vi "ReadATEQData.vi"(11 "Chaîne":string) -> (0 "Prg number":string, 1 "Valeur":i32, 2 "result":string, 3 "Status":string)   [LabVIEW 2020]
uses:
  <vilib>/regexp/Match Regular Expression.xnode
panel:
  # "<20>:(AL):PRESSION HAUTE\n<30>:(DR):-126 Pa\n<30>:(DT):2 Pa\n<30>:(DR):-10 Pa\n<30>:(PB):1 Pa\n<30>:(PB):1 Pa\n<30>:(PB):-2 Pa\n<30>:(DR):-197 Pa\n^C"
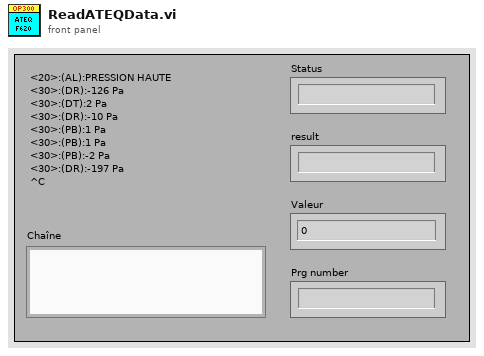
[diagram p1: front panel]
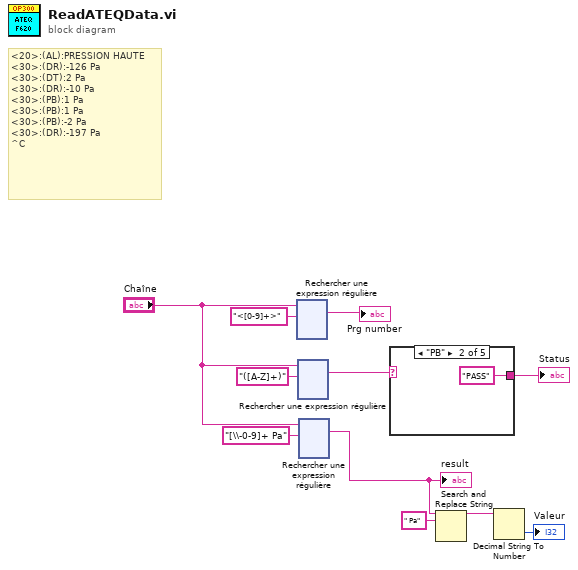
[diagram p0: block diagram]
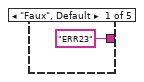
[diagram p2: hidden frame]
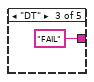
[diagram p3: hidden frame]
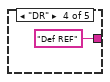
[diagram p4: hidden frame]
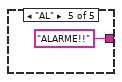
[diagram p5: hidden frame]
diagram:
  # "<20>:(AL):PRESSION HAUTE\n<30>:(DR):-126 Pa\n<30>:(DT):2 Pa\n<30>:(DR):-10 Pa\n<30>:(PB):1 Pa\n<30>:(PB):1 Pa\n<30>:(PB):-2 Pa\n<30>:(DR):-197 Pa\n^C"
  n1 = xnode "Rechercher une expression régulière"("chaîne en entrée"="Chaîne", "expression régulière"="<[0-9]+>") -> ("toute l'expression"=→"Prg number":string)  [unwired: 4 in, 4 out]
  n2 = xnode "Rechercher une expression régulière"("chaîne en entrée"="Chaîne", "expression régulière"="([A-Z]+)") -> ("toute l'expression"=w8:string)  [unwired: 4 in, 4 out]
  n3 = xnode "Rechercher une expression régulière"("chaîne en entrée"="Chaîne", "expression régulière"="[\\-0-9]+ Pa") -> ("toute l'expression"=w4:string)  [unwired: 4 in, 4 out]
  "result" <- w4
  n4 = case shown="\"PB\"" w8 {
    tunnel: ["ERR23" "PASS" "FAIL" "Def REF" "ALARME!!"] -> w7
    frame "Faux", Default {
    }
    frame "PB" {
    }
    frame "DT" {
    }
    frame "DR" {
    }
    frame "AL" {
    }
  }
  "Status" <- w7
  n5 = Search and Replace String ("Rechercher et remplacer une chaîne")(input string=w4, search string=" Pa" ("chaîne recherchée")) -> (result string=w2:string)  [unwired: 6 in, 3 out]
  n6 = Decimal String To Number ("Chaîne décimale en nombre")(string=w2) -> (number=→"Valeur":i32)  [unwired: 2 in, 1 out]
